vi "Get_Amplitude.vi"(1 "Data QY":string, 2 "Data QX":string) -> (0 "Numeric":dbl)   [LabVIEW 2010]
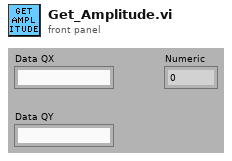
[diagram p1: front panel]
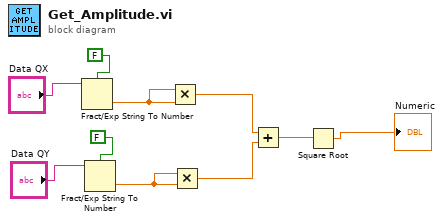
[diagram p0: block diagram]
diagram:
  n1 = Fract/Exp String To Number(use system decimal point (T)=FALSE, string="Data QX") -> (number=w5:dbl)  [unwired: 2 in, 1 out]
  n2 = Fract/Exp String To Number(use system decimal point (T)=FALSE, string="Data QY") -> (number=w6:dbl)  [unwired: 2 in, 1 out]
  n3 = Multiply(x=w5, y=w5) -> (x*y=w7:dbl)
  n4 = Multiply(x=w6, y=w6) -> (x*y=w8:dbl)
  n5 = Add(x=w7, y=w8) -> (x+y=w9:dbl)
  n6 = Square Root(x=w9) -> (sqrt(x)=→"Numeric":dbl)
